vi "Reduced Time curtail and pf.vi"() -> ()   [LabVIEW 2018]
uses:
  749368e9-8a13-4457-ac74-086f0bb157c2.vi
  1ca09a49-d2c4-4d2a-8422-a7731fce5b7b.vi
  a7e399ce-82dc-48aa-a6e2-ac362b8dfa23.vi
  75f83434-2c83-437c-aa7d-48cbf84b3d36.vi
  6cf8bfcf-bab5-4fe0-9dd9-fe191ab04daa.vi
  010fc5d1-faf8-4fdd-ade0-65e49e8fa1d8.vi
  <vilib>/Plasmionique/MB Master/MB_Master_TCP/MB_Master_TCP.lvclass
  C:/Program Files (x86)/National Instruments/LabVIEW 2018/vi.lib/Plasmionique/MB Master/MB_Master/MB_Master.lvclass
  <vilib>/Plasmionique/MB Master/MB Master.lvlib
panel:
  out "Setup Complete":bool
  in  "Inverter IP Address":string
  out "Setup Runtime (s)":u32
  in  "Setup Curtailment and Power Factor":bool
  out "Curtailment Complete":bool
  out "Power Factor Complete":bool
  out "Power Factor Runtime (s)":u32
  out "Curtailment Runtime (s)":u32
  in  "Stop Button":bool
  in  "Send Power Factor":bool
  in  "Send Curtailment":bool
  in  "Curtailment % (28-100)":u16
  in  "Power Factor Setpoint":i32
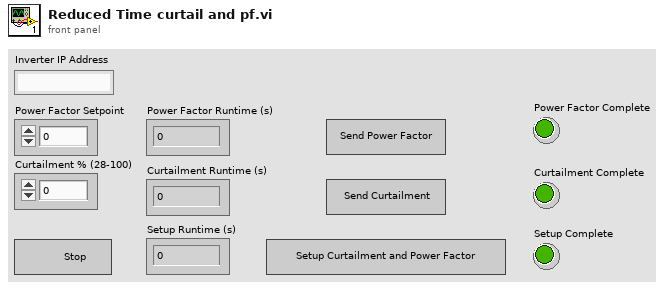
[diagram p1: front panel]
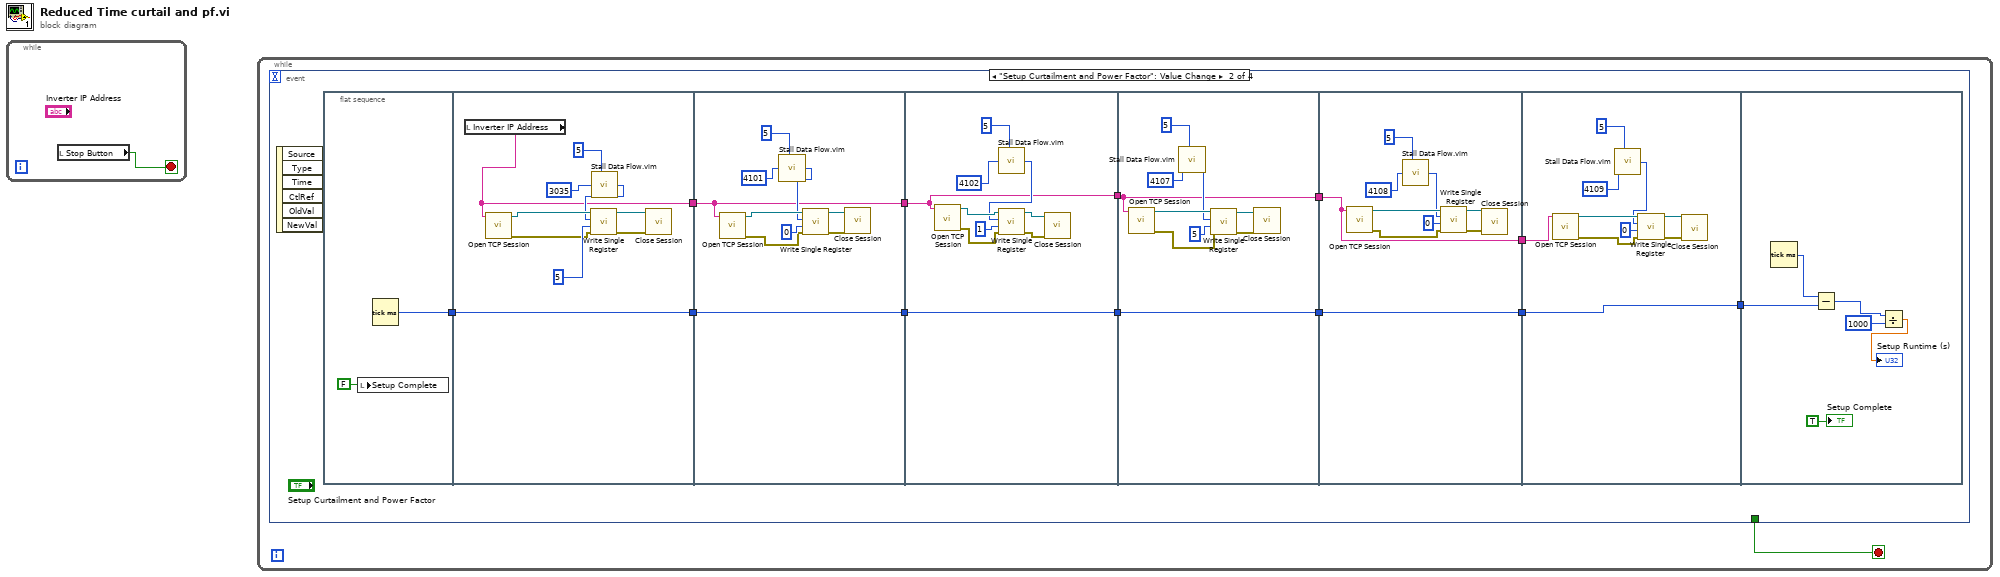
[diagram p0: block diagram]
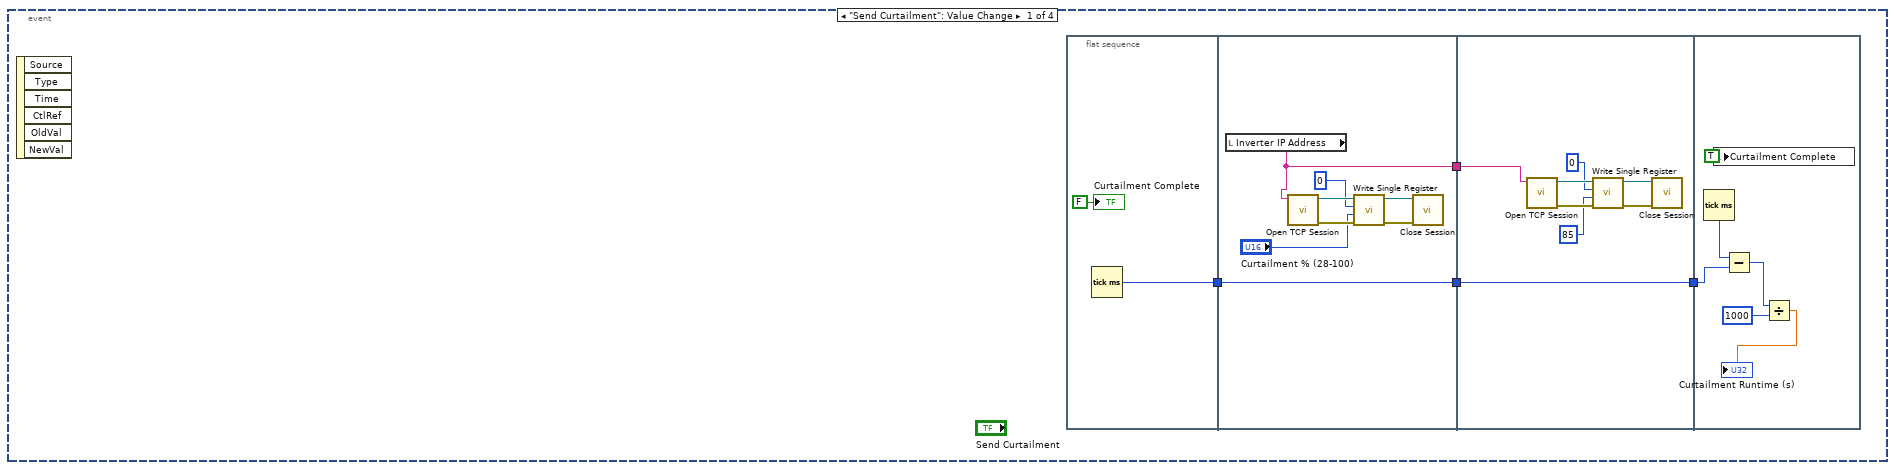
[diagram p2: hidden frame]
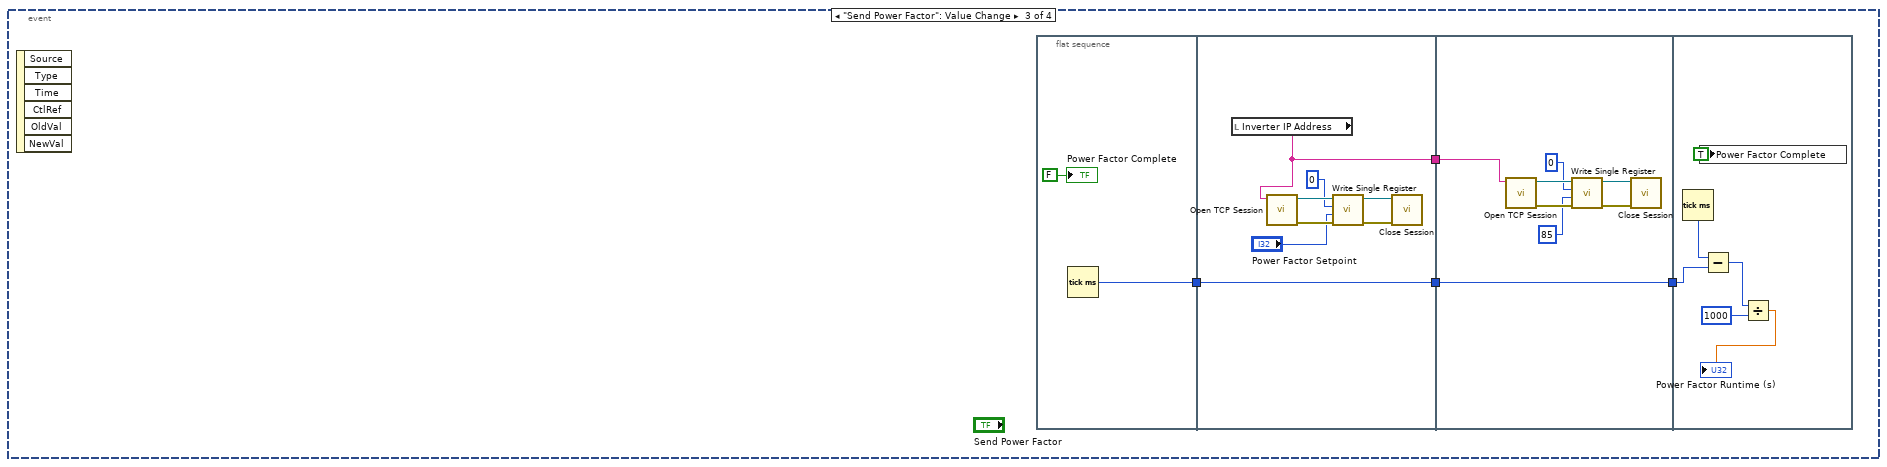
[diagram p3: hidden frame]
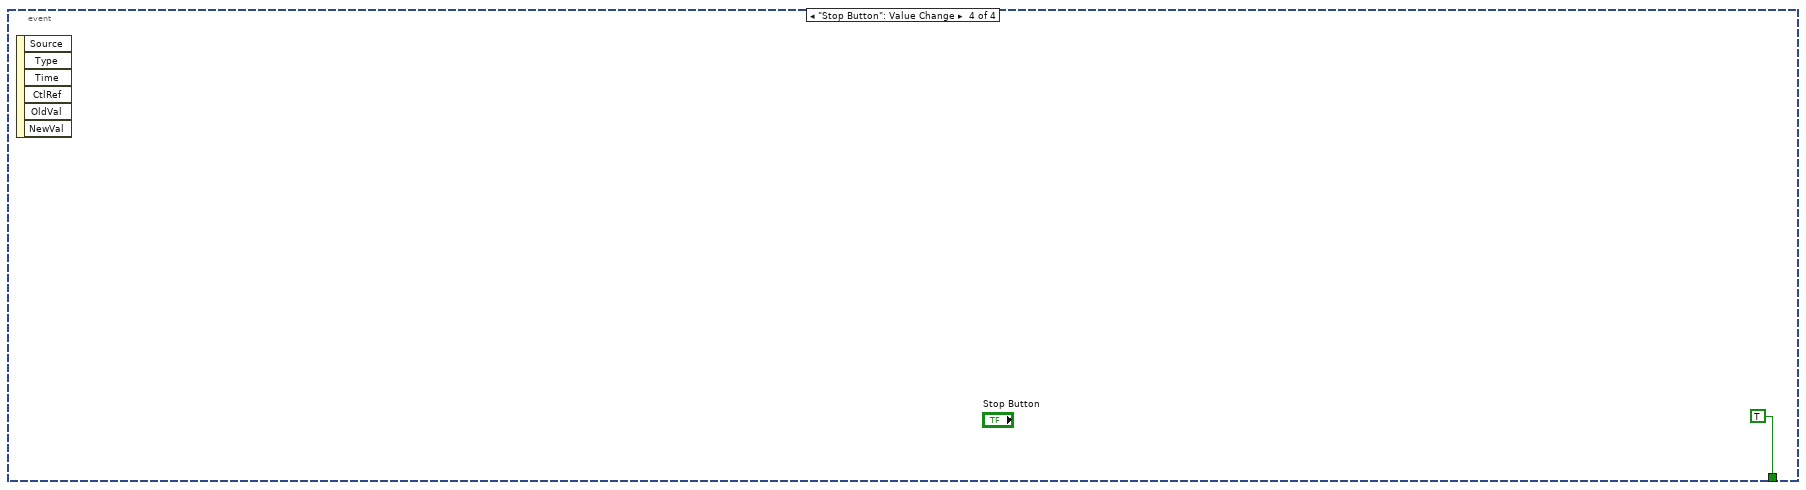
[diagram p4: hidden frame]
diagram:
  n1 = while {
    stop <- w1 stop-if-true
    n2 = local read "Stop Button"() -> (w1:bool)
  }
  n3 = while {
    stop <- w2 stop-if-true
    n4 = event shown="[1] \"Setup Curtailment and Power Factor\": Value Change" {
      selector: _ -> [_ _ _ _]
      dyn-events: _ -> [_ _ _ _]
      timeout: _ -> [_ _ _ _]
      tunnel: [_ _ _ TRUE] -> w2
      event "Send Curtailment": Value Change {
        n5 = event-data() -> ()  [unwired: 1 in, 6 out]
        n6 = flat-sequence {
          tunnel: [w8] -> w6
          tunnel: w6 -> [w11]
          tunnel: [w11] -> w4
          tunnel: [w9] -> w3
          tunnel: [w24] -> w5
          tunnel: w4 -> [w24]
          tunnel: w3 -> [w17]
          tunnel: w5 -> [w29]
          frame #0 {
            n7 = Tick Count (ms)() -> (millisecond timer value=w8:u32)
            "Curtailment Complete" <- FALSE ("Curtailment Sent")
          }
          frame #1 {
            n8 = local read "Inverter IP Address"() -> (w9:string)
            n9 = call <vilib>:"Open TCP Session.vi"("IP Address"=w9) -> ("error out"=w14:errorcluster, "MB_TCP session"=w16:refnum<class "MB_Master_TCP.lvclass">)  [unwired: 9 in]
            n10 = call <vilib>:"Write Single Register.vi"("error in (no error)"=w14, "value"="Curtailment % (28-100)", "address"=u16 0, "MB session in"=w16) -> ("error out"=w13:errorcluster, "MB session out"=w12:refnum<class "MB_Master_TCP.lvclass">)  [unwired: 6 in]
            n11 = call-dynamic "Close Session.vi"("error in (no error)"=w13, "MB TCP session"=w12) -> ()  [unwired: 9 in, 1 out]
          }
          frame #2 {
            n12 = call <vilib>:"Open TCP Session.vi"("IP Address"=w17) -> ("error out"=w21:errorcluster, "MB_TCP session"=w23:refnum<class "MB_Master_TCP.lvclass">)  [unwired: 9 in]
            n13 = call <vilib>:"Write Single Register.vi"("error in (no error)"=w21, "value"=u16 85, "address"=u16 0, "MB session in"=w23) -> ("error out"=w20:errorcluster, "MB session out"=w19:refnum<class "MB_Master_TCP.lvclass">)  [unwired: 6 in]
            n14 = call-dynamic "Close Session.vi"("error in (no error)"=w20, "MB TCP session"=w19) -> ()  [unwired: 9 in, 1 out]
          }
          frame #3 {
            n15 = Tick Count (ms)() -> (millisecond timer value=w30:u32)
            n16 = local write "Curtailment Complete"(TRUE ("Curtailment Sent")) -> ()
            n17 = Subtract(x=w30, y=w29) -> (x-y=w28:u32)
            n18 = Divide(x=w28, y=u32 1000) -> (x/y=→"Curtailment Runtime (s)":dbl)
          }
        }
      }
      event "Setup Curtailment and Power Factor": Value Change {
        n19 = event-data() -> ()  [unwired: 1 in, 6 out]
        n20 = flat-sequence {
          tunnel: [w44] -> w42
          tunnel: [w46] -> w41
          tunnel: w42 -> [w46]
          tunnel: [w45] -> w40
          tunnel: [w56] -> w39
          tunnel: w41 -> [w56]
          tunnel: w40 -> [w55]
          tunnel: [w55] -> w38
          tunnel: [w66] -> w37
          tunnel: w39 -> [w66]
          tunnel: w38 -> [w65]
          tunnel: [w65] -> w36
          tunnel: [w76] -> w35
          tunnel: w37 -> [w76]
          tunnel: w36 -> [w75]
          tunnel: [w75] -> w34
          tunnel: [w86] -> w33
          tunnel: w35 -> [w86]
          tunnel: w34 -> [w85]
          tunnel: [w85] -> w32
          tunnel: w33 -> [w95]
          tunnel: w32 -> [w96]
          tunnel: [w95] -> w31
          tunnel: w31 -> [w109]
          frame #0 {
            n21 = local write "Setup Complete"(FALSE ("Setup Complete")) -> ()
            n22 = Tick Count (ms)() -> (millisecond timer value=w44:u32)
          }
          frame #1 {
            n23 = local read "Inverter IP Address"() -> (w45:string)
            n24 = call <vilib>:"Open TCP Session.vi"("IP Address"=w45) -> ("error out"=w51:errorcluster, "MB_TCP session"=w50:refnum<class "MB_Master_TCP.lvclass">)  [unwired: 9 in]
            n25 = call "Stall Data Flow.vim"("value in"=u16 3035 ("address"), "milliseconds to wait"=u32 5) -> ("value out"=w47:u16)  [unwired: 1 out]
            n26 = call <vilib>:"Write Single Register.vi"("error in (no error)"=w51, "value"=u16 5, "address"=w47, "MB session in"=w50) -> ("error out"=w52:errorcluster, "MB session out"=w53:refnum<class "MB_Master_TCP.lvclass">)  [unwired: 6 in]
            n27 = call-dynamic "Close Session.vi"("error in (no error)"=w52, "MB TCP session"=w53) -> ()  [unwired: 9 in, 1 out]
          }
          frame #2 {
            n28 = call <vilib>:"Open TCP Session.vi"("IP Address"=w55) -> ("error out"=w62:errorcluster, "MB_TCP session"=w63:refnum<class "MB_Master_TCP.lvclass">)  [unwired: 9 in]
            n29 = call "Stall Data Flow.vim"("value in"=u16 4101 ("address"), "milliseconds to wait"=u32 5) -> ("value out"=w57:u16)  [unwired: 1 out]
            n30 = call <vilib>:"Write Single Register.vi"("error in (no error)"=w62, "value"=u16 0, "address"=w57, "MB session in"=w63) -> ("error out"=w61:errorcluster, "MB session out"=w60:refnum<class "MB_Master_TCP.lvclass">)  [unwired: 6 in]
            n31 = call-dynamic "Close Session.vi"("error in (no error)"=w61, "MB TCP session"=w60) -> ()  [unwired: 9 in, 1 out]
          }
          frame #3 {
            n32 = call <vilib>:"Open TCP Session.vi"("IP Address"=w65) -> ("error out"=w70:errorcluster, "MB_TCP session"=w73:refnum<class "MB_Master_TCP.lvclass">)  [unwired: 9 in]
            n33 = call "Stall Data Flow.vim"("value in"=u16 4102 ("address"), "milliseconds to wait"=u32 5) -> ("value out"=w67:u16)  [unwired: 1 out]
            n34 = call <vilib>:"Write Single Register.vi"("error in (no error)"=w70, "value"=u16 1, "address"=w67, "MB session in"=w73) -> ("error out"=w72:errorcluster, "MB session out"=w71:refnum<class "MB_Master_TCP.lvclass">)  [unwired: 6 in]
            n35 = call-dynamic "Close Session.vi"("error in (no error)"=w72, "MB TCP session"=w71) -> ()  [unwired: 9 in, 1 out]
          }
          frame #4 {
            n36 = call <vilib>:"Open TCP Session.vi"("IP Address"=w75) -> ("error out"=w80:errorcluster, "MB_TCP session"=w83:refnum<class "MB_Master_TCP.lvclass">)  [unwired: 9 in]
            n37 = call "Stall Data Flow.vim"("value in"=u16 4107 ("address"), "milliseconds to wait"=u32 5) -> ("value out"=w77:u16)  [unwired: 1 out]
            n38 = call <vilib>:"Write Single Register.vi"("error in (no error)"=w80, "value"=u16 5, "address"=w77, "MB session in"=w83) -> ("error out"=w82:errorcluster, "MB session out"=w81:refnum<class "MB_Master_TCP.lvclass">)  [unwired: 6 in]
            n39 = call-dynamic "Close Session.vi"("error in (no error)"=w82, "MB TCP session"=w81) -> ()  [unwired: 9 in, 1 out]
          }
          frame #5 {
            n40 = call <vilib>:"Open TCP Session.vi"("IP Address"=w85) -> ("error out"=w90:errorcluster, "MB_TCP session"=w93:refnum<class "MB_Master_TCP.lvclass">)  [unwired: 9 in]
            n41 = call "Stall Data Flow.vim"("value in"=u16 4108 ("address"), "milliseconds to wait"=u32 5) -> ("value out"=w88:u16)  [unwired: 1 out]
            n42 = call <vilib>:"Write Single Register.vi"("error in (no error)"=w90, "value"=u16 0, "address"=w88, "MB session in"=w93) -> ("error out"=w92:errorcluster, "MB session out"=w91:refnum<class "MB_Master_TCP.lvclass">)  [unwired: 6 in]
            n43 = call-dynamic "Close Session.vi"("error in (no error)"=w92, "MB TCP session"=w91) -> ()  [unwired: 9 in, 1 out]
          }
          frame #6 {
            n44 = call <vilib>:"Open TCP Session.vi"("IP Address"=w96) -> ("error out"=w102:errorcluster, "MB_TCP session"=w103:refnum<class "MB_Master_TCP.lvclass">)  [unwired: 9 in]
            n45 = call "Stall Data Flow.vim"("value in"=u16 4109 ("address"), "milliseconds to wait"=u32 5) -> ("value out"=w97:u16)  [unwired: 1 out]
            n46 = call <vilib>:"Write Single Register.vi"("error in (no error)"=w102, "value"=u16 0, "address"=w97, "MB session in"=w103) -> ("error out"=w100:errorcluster, "MB session out"=w101:refnum<class "MB_Master_TCP.lvclass">)  [unwired: 6 in]
            n47 = call-dynamic "Close Session.vi"("error in (no error)"=w100, "MB TCP session"=w101) -> ()  [unwired: 9 in, 1 out]
          }
          frame #7 {
            n48 = Tick Count (ms)() -> (millisecond timer value=w110:u32)
            n49 = Subtract(x=w110, y=w109) -> (x-y=w108:u32)
            n50 = Divide(x=w108, y=u32 1000) -> (x/y=→"Setup Runtime (s)":dbl)
            "Setup Complete" <- TRUE ("Setup Complete")
          }
        }
      }
      event "Send Power Factor": Value Change {
        n51 = event-data() -> ()  [unwired: 1 in, 6 out]
        n52 = flat-sequence {
          tunnel: [w116] -> w114
          tunnel: w114 -> [w119]
          tunnel: [w119] -> w113
          tunnel: [w117] -> w111
          tunnel: [w132] -> w112
          tunnel: w113 -> [w132]
          tunnel: w111 -> [w125]
          tunnel: w112 -> [w137]
          frame #0 {
            n53 = Tick Count (ms)() -> (millisecond timer value=w116:u32)
            "Power Factor Complete" <- FALSE ("Curtailment Sent")
          }
          frame #1 {
            n54 = local read "Inverter IP Address"() -> (w117:string)
            n55 = call <vilib>:"Open TCP Session.vi"("IP Address"=w117) -> ("error out"=w122:errorcluster, "MB_TCP session"=w124:refnum<class "MB_Master_TCP.lvclass">)  [unwired: 9 in]
            n56 = call <vilib>:"Write Single Register.vi"("error in (no error)"=w122, "value"="Power Factor Setpoint", "address"=u16 0, "MB session in"=w124) -> ("error out"=w121:errorcluster, "MB session out"=w120:refnum<class "MB_Master_TCP.lvclass">)  [unwired: 6 in]
            n57 = call-dynamic "Close Session.vi"("error in (no error)"=w121, "MB TCP session"=w120) -> ()  [unwired: 9 in, 1 out]
          }
          frame #2 {
            n58 = call <vilib>:"Open TCP Session.vi"("IP Address"=w125) -> ("error out"=w129:errorcluster, "MB_TCP session"=w131:refnum<class "MB_Master_TCP.lvclass">)  [unwired: 9 in]
            n59 = call <vilib>:"Write Single Register.vi"("error in (no error)"=w129, "value"=u16 85, "address"=u16 0, "MB session in"=w131) -> ("error out"=w128:errorcluster, "MB session out"=w127:refnum<class "MB_Master_TCP.lvclass">)  [unwired: 6 in]
            n60 = call-dynamic "Close Session.vi"("error in (no error)"=w128, "MB TCP session"=w127) -> ()  [unwired: 9 in, 1 out]
          }
          frame #3 {
            n61 = Tick Count (ms)() -> (millisecond timer value=w138:u32)
            n62 = local write "Power Factor Complete"(TRUE ("Curtailment Sent")) -> ()
            n63 = Subtract(x=w138, y=w137) -> (x-y=w136:u32)
            n64 = Divide(x=w136, y=u32 1000) -> (x/y=→"Power Factor Runtime (s)":dbl)
          }
        }
      }
      event "Stop Button": Value Change {
        n65 = event-data() -> ()  [unwired: 1 in, 6 out]
      }
    }
  }
